vi "Update Property.vi"(8 "error in (no error)":errorcluster, 9 "Value":variant, 10 "Name":string, 11 "DoublePanel in":refnum<class "DoublePanel.lvclass">) -> (0 "error out":errorcluster, 3 "DoublePanel out":refnum<class "DoublePanel.lvclass">)   [LabVIEW 2020, in "Conditum-Tools.lvlib" / "DoublePanel.lvclass"]
uses:
  DoublePanel.lvclass
  DoublePanel.lvclass/DoublePanel.ctl
  Conditum-Clone/Columns/Double/Double.lvclass
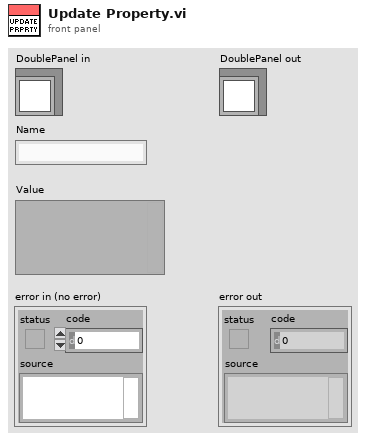
[diagram p1: front panel]
types:
  T1 = typedef "Conditu2.lvlib/Columns.lvlib/Double.lvclass/Definition.ctl" = cluster{"Default":dbl}
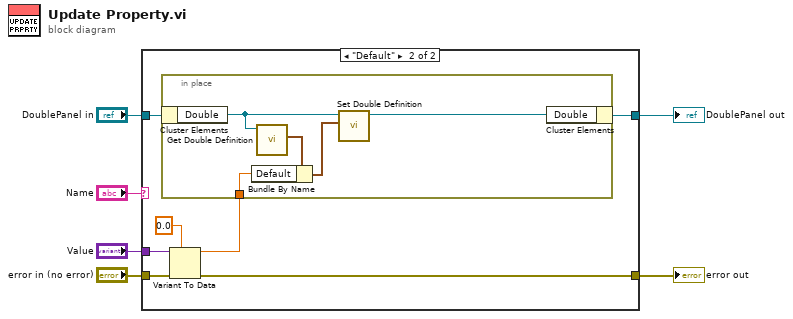
[diagram p0: block diagram]
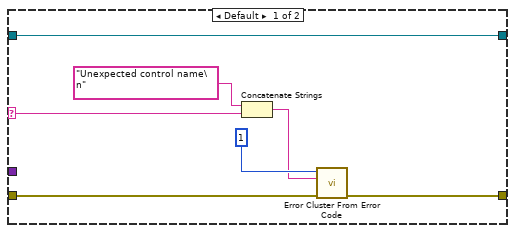
[diagram p2: hidden frame]
diagram:
  n1 = case shown="\"Default\"" "Name" {
    selector: "Name" -> [w9 _]
    tunnel: "Value" -> [_ w20]
    tunnel: "DoublePanel in" -> [w7 w16]
    tunnel: "error in (no error)" -> [w13 w18]
    tunnel: [w12 w17] -> w3
    tunnel: [w7 w14] -> w5
    frame Default {
      n2 = Concatenate Strings("Unexpected control name\n" ("format string"), w9) -> (w8:string)
      n3 = call <vilib>:"Error Cluster From Error Code.vi"("error in (no error)"=w13, "error message (\"\")"=w8, "error code (0)"=1) -> ("error out"=w12:errorcluster)  [unwired: 6 in]
    }
    frame "Default" {
      n4 = Variant To Data(error in=w18, type=0.0, Variant=w20) -> (data=w15:dbl, error out=w17:errorcluster)
      n5 = in-place {
        in-place-border: w15 -> [w24]
        n6 = in-place-cluster #1(w16) -> ("Double"=w23:refnum<class "Double.lvclass">)
        n7 = call "Get Double Definition.vi"("Double in"=w23) -> ("Definition"=w25:T1)  [unwired: 10 in]
        n8 = Bundle By Name(cluster=w25, "Default"=w24) -> (w22:T1)
        n9 = call "Set Double Definition.vi"("Double Definition"=w22, "Double in"=w23) -> ("Double out"=w21:refnum<class "Double.lvclass">)  [unwired: 9 in]
        n10 = in-place-cluster #1("Double"=w21) -> (w14:refnum<class "DoublePanel.lvclass">)
      }
    }
  }
  "error out" <- w3
  "DoublePanel out" <- w5
